vi "MDAQ_ArrayHelp.vi"(7 "Sum":u32, 10 "Input Cluster":T2 {"CV"."Temperature Array" scale=0.0..100.0}, 11 "Concurrent CV Arrays":T1) -> (2 "Output Cluster":T2 {"CV"."Temperature Array" scale=0.0..100.0}, 3 "Concurrent CV Arrays Out":T1)   [LabVIEW 2021]
uses:
  GUI_Def.ctl
  Mode_Enum.ctl
  Array_Cluster.ctl
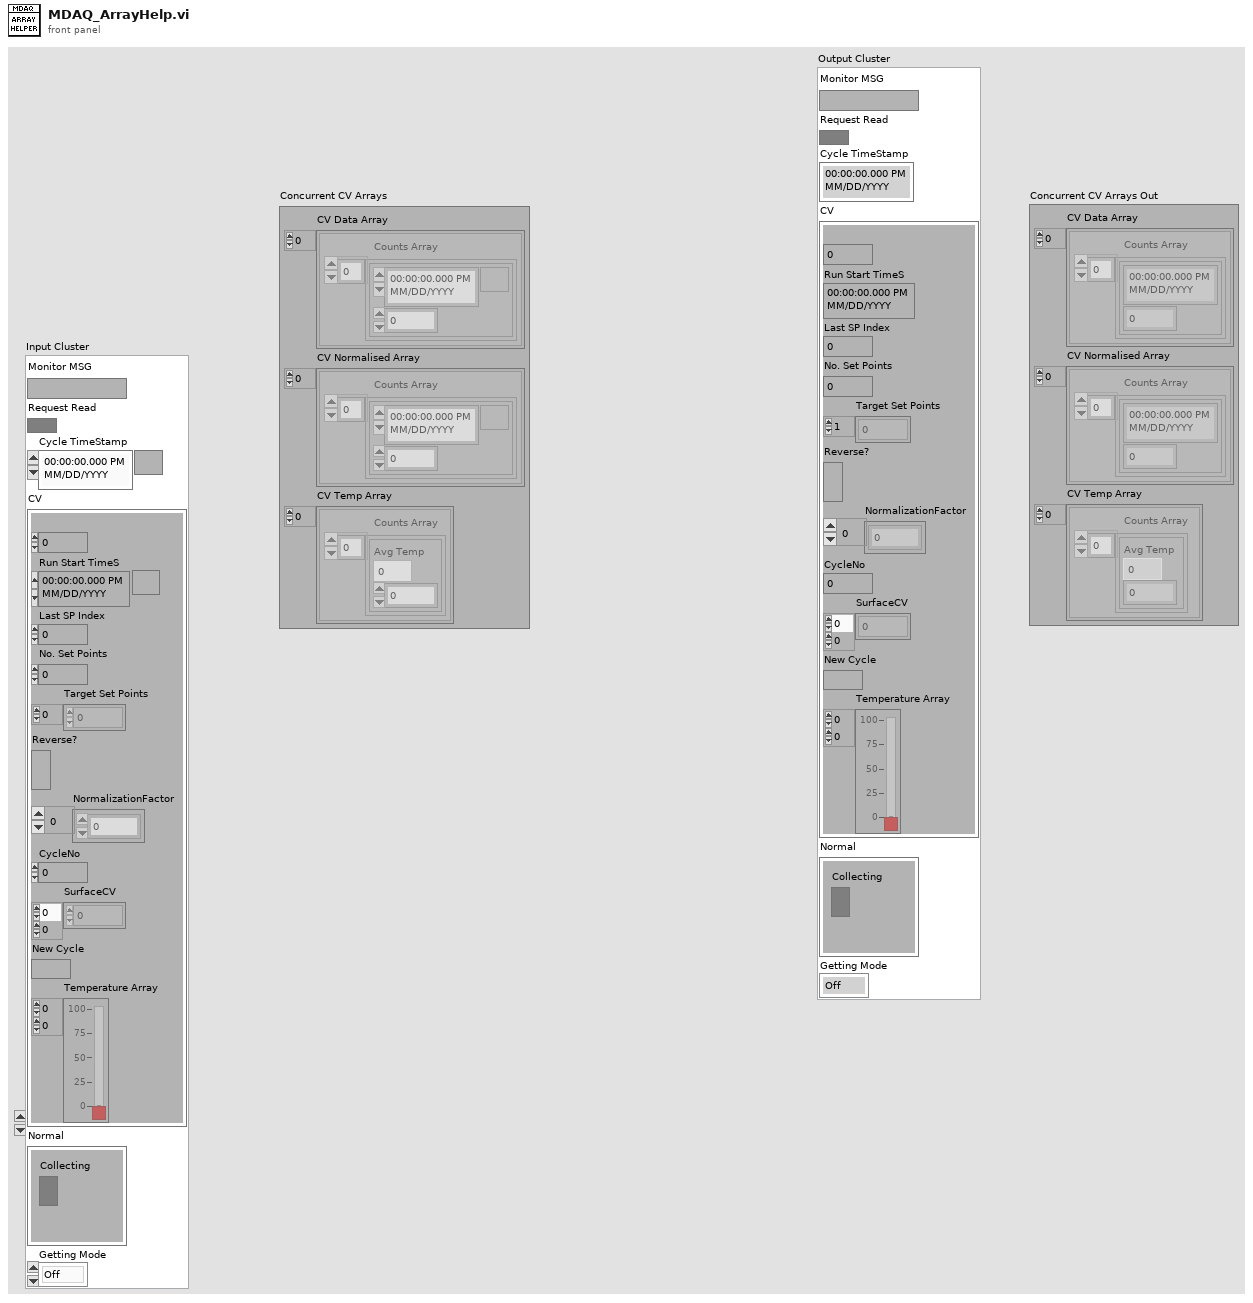
[diagram p1: front panel]
types:
  T1 = typedef "Array_Cluster.ctl" = cluster{"CV Data Array":cluster{"Counts Array":cluster{timestamp, i32}[]}[], "CV Normalised Array":cluster{"Counts Array":cluster{timestamp, dbl}[]}[], "CV Temp Array":cluster{"Counts Array":cluster{"Avg Temp":dbl, dbl}[]}[]}
  T2 = typedef "GUI_Def.ctl" = cluster{"Monitor MSG":string, "Request Read":bool, "Cycle TimeStamp":timestamp, "CV":cluster{"Set Point Index":u32, "Run Start TimeS":timestamp, "Last SP Index":u32, "No. Set Points":u32, "Target Set Points":i32[], "Reverse?":bool, "NormalizationFactor":i32[], "CycleNo":i32, "SurfaceCV":dbl[][], "New Cycle":bool, "Temperature Array":dbl[][]}, "Normal":cluster{"Collecting":bool}, "Getting Mode":T3}
  T3 = typedef "Mode_Enum.ctl" = enum16{"Off", "Normal", "CV+Temp", "CV"}
  T4 = cluster{"Counts Array":cluster{"Avg Temp":dbl, dbl}[]}[]
  T5 = cluster{"Counts Array":cluster{timestamp, i32}[]}[]
  T6 = cluster{"Counts Array":cluster{"Avg Temp":dbl, dbl}[]}
  T7 = cluster{"Counts Array":cluster{timestamp, i32}[]}
  T8 = cluster{"seconds since 1Jan1904":timestamp, "Sum":u32}
  T9 = cluster{"Counts Array":cluster{timestamp, dbl}[]}[]
  T10 = cluster{"Counts Array":cluster{timestamp, dbl}[]}
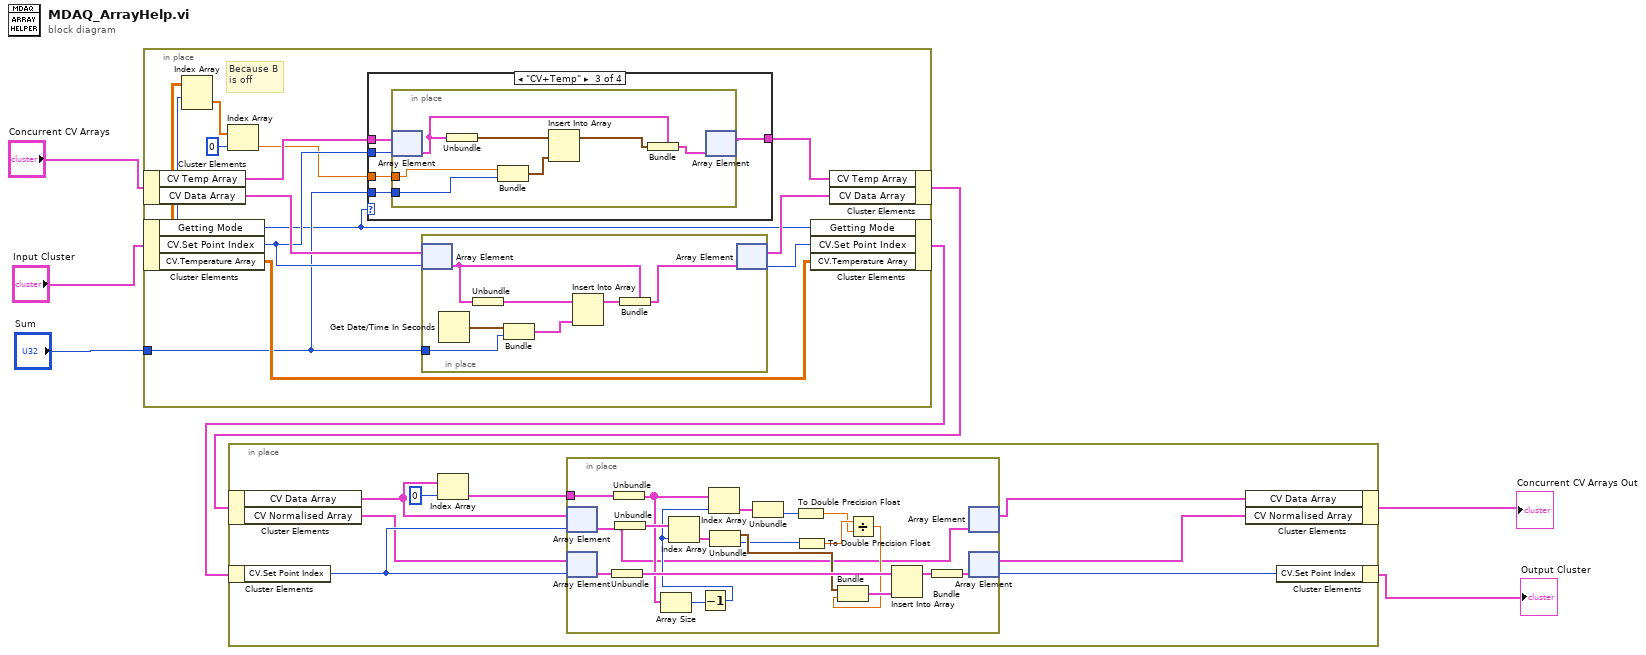
[diagram p0: block diagram]
diagram:
  n1 = in-place {
    in-place-border: "Sum" -> [w9]
    # "Because B\nis off"
    n2 = in-place-cluster #1("Concurrent CV Arrays") -> ("CV Temp Array"=w13:T4, "CV Data Array"=w18:T5)
    n3 = in-place-cluster #2("Input Cluster") -> ("Getting Mode"=w8:T3, "CV.Set Point Index"=w12:u32, "CV.Temperature Array"=w16:dbl[][])
    n4 = Index Array(array=w16, index (row)=w12) -> (element=w15:dbl[])  [unwired: 1 in]
    n5 = Index Array(array=w15, index=0) -> (element=w11:dbl)
    n6 = case shown="\"CV+Temp\"" w8 {
      tunnel: w13 -> [w20 w21 w26 w34]
      tunnel: w12 -> [_ _ w25 _]
      tunnel: w11 -> [_ _ w24 _]
      tunnel: [w20 w21 w23 w34] -> w10
      tunnel: w9 -> [_ _ w22 _]
      frame "Off", Default {
      }
      frame "Normal" {
      }
      frame "CV+Temp" {
        n7 = in-place {
          in-place-border: w24 -> [w29]
          in-place-border: w22 -> [w27]
          n8 = in-place-array #3(w26, w25) -> (w28:T6)
          n9 = Unbundle(w28) -> ("Counts Array"=w33:cluster{"Avg Temp":dbl, dbl}[])
          n10 = Bundle("Thermometer"=w29, "Sum"=w27) -> (w32:cluster{"Thermometer":dbl, "Sum":u32})  [unwired: 1 in]
          n11 = Insert Into Array(array=w33, new element=w32) -> (w31:cluster{"Avg Temp":dbl, dbl}[])  [unwired: 1 in]
          n12 = Bundle(cluster=w28, "Counts Array"=w31) -> (w30:T6)
          n13 = in-place-array #3(w30) -> (w23:T4)  [unwired: 1 out]
        }
      }
      frame "CV" {
      }
    }
    n14 = in-place {
      in-place-border: w9 -> [w35]
      n15 = in-place-array #4(w18, w12) -> (w39:T7)
      n16 = Get Date/Time In Seconds() -> (seconds since 1Jan1904=w41:timestamp)
      n17 = Unbundle(w39) -> ("Counts Array"=w38:cluster{timestamp, i32}[])
      n18 = Bundle("seconds since 1Jan1904"=w41, "Sum"=w35) -> (w36:T8)  [unwired: 1 in]
      n19 = Insert Into Array(array=w38, new element=w36) -> (w37:cluster{timestamp, i32}[])  [unwired: 1 in]
      n20 = Bundle(cluster=w39, "Counts Array"=w37) -> (w40:T7)
      n21 = in-place-array #4(w40) -> (w17:T5, w19:i32)
    }
    n22 = in-place-cluster #2("Getting Mode"=w8, "CV.Set Point Index"=w19, "CV.Temperature Array"=w16) -> (w5:T2)
    n23 = in-place-cluster #1("CV Temp Array"=w10, "CV Data Array"=w17) -> (w2:T1)
  }
  n24 = in-place {
    n25 = in-place-cluster #5(w2) -> ("CV Data Array"=w45:T5, "CV Normalised Array"=w44:T9)
    n26 = in-place-cluster #6(w5) -> ("CV.Set Point Index"=w48:u32)
    n27 = Index Array(array=w45, index=0) -> (element=w47:T7)
    n28 = in-place {
      in-place-border: w47 -> [w68]
      n29 = in-place-array #7(w45, w48) -> (w53:T7)
      n30 = in-place-array #8(w44, w48) -> (w52:T10)
      n31 = Unbundle(w52) -> ("Counts Array"=w65:cluster{timestamp, dbl}[])
      n32 = Unbundle(w68) -> ("Counts Array"=w56:cluster{timestamp, i32}[])
      n33 = Unbundle(w53) -> ("Counts Array"=w67:cluster{timestamp, i32}[])
      n34 = Array Size(array=w56) -> (size(s)=w55:i32)
      n35 = Decrement(x=w55) -> (x-1=w54:i32)
      n36 = Index Array(array=w67, index=w54) -> (element=w66:cluster{timestamp, i32})
      n37 = Index Array(array=w56, index=w54) -> (element=w62:cluster{timestamp, i32})
      n38 = Unbundle(w66) -> (w63:timestamp, w60:i32)
      n39 = Unbundle(w62) -> (w61:i32)  [unwired: 1 out]
      n40 = To Double Precision Float(number=w61) -> (double precision float=w58:dbl)
      n41 = To Double Precision Float(number=w60) -> (double precision float=w59:dbl)
      n42 = Divide(x=w59, y=w58) -> (x/y=w57:dbl)
      n43 = Bundle(w63, w57) -> (w64:cluster{timestamp, dbl})  [unwired: 1 in]
      n44 = Insert Into Array(array=w65, new element=w64) -> (w51:cluster{timestamp, dbl}[])  [unwired: 1 in]
      n45 = Bundle("Counts Array"=w51) -> (w50:T10)  [unwired: 1 in]
      n46 = in-place-array #7(w53) -> (w43:T5)  [unwired: 1 out]
      n47 = in-place-array #8(w50) -> (w42:T9, w46:i32)
    }
    n48 = in-place-cluster #5("CV Data Array"=w43, "CV Normalised Array"=w42) -> (→"Concurrent CV Arrays Out":T1)
    n49 = in-place-cluster #6("CV.Set Point Index"=w46) -> (→"Output Cluster":T2)
  }
